vi "PQ setpoint hold.vi"(7 "VF mode":bool, 8 "Qmeas_ES":sgl, 11 "Pmeas_ES":sgl) -> (0 "Qhold":sgl, 3 "Phold":sgl)   [LabVIEW 2015]
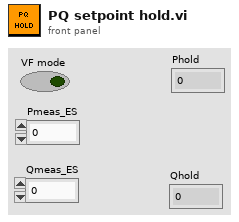
[diagram p1: front panel]
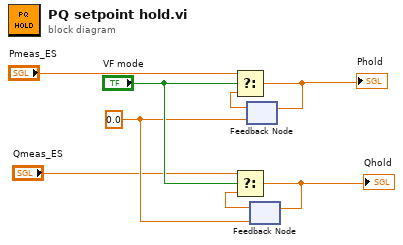
[diagram p0: block diagram]
diagram:
  w7 = sgl 0.0 ("Pmeas_ES")
  n1 = feedback #1(w7) -> (w4:sgl)
  n2 = Select(t="Pmeas_ES", s="VF mode", f=w4) -> (s? t:f=w3:sgl)
  "Phold" <- w3
  n3 = feedback-in #1(w3) -> ()
  n4 = feedback #2(w7) -> (w6:sgl)
  n5 = Select(t="Qmeas_ES", s="VF mode", f=w6) -> (s? t:f=w5:sgl)
  "Qhold" <- w5
  n6 = feedback-in #2(w5) -> ()
